vi "CheckMove.vi"(8 "error in":errorcluster caption="entrée d'erreur", 10 "Go to (mm)":dbl[](array[numeric]) format="%.6f", 11 "Limits":dbl[](array[numeric]) format="%.6f") -> (0 "error out":errorcluster caption="sortie d'erreur", 3 "Validated!":bool)   [LabVIEW 2026]
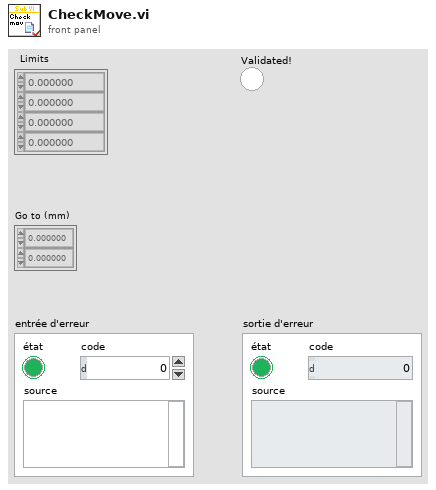
[diagram p1: front panel]
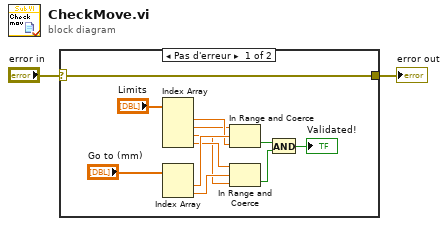
[diagram p0: block diagram]
diagram:
  n1 = case shown="Pas d'erreur" "error in" {
    selector: "error in" -> [w13 w15]
    tunnel: [w13 w15] -> w1
    frame No Error {
      n2 = Index Array(array="Limits") -> (element #1=w9:dbl, element #2=w8:dbl, element #3=w6:dbl, element #4=w7:dbl)  [unwired: 4 in]
      n3 = Index Array(array="Go to (mm)") -> (element #1=w12:dbl, element #2=w11:dbl)  [unwired: 2 in]
      n4 = In Range and Coerce(upper limit=w8, x=w12, lower limit=w9) -> (In Range?=w5:bool)  [unwired: 1 out]
      n5 = In Range and Coerce(upper limit=w7, x=w11, lower limit=w6) -> (In Range?=w4:bool)  [unwired: 1 out]
      n6 = And(x=w5, y=w4) -> (x .and. y?=→"Validated!":bool)
    }
    frame Error {
    }
  }
  "error out" <- w1
